vi "Calculate_fit_offset.vi"(0 "baseline1":dbl[](array[numeric]), 3 "baseline2":dbl[](array[numeric])) -> (6 "Peak_ch1":dbl format="%#_6f", 7 "Std_dev_ch1":dbl format="%#_6f", 8 "Peak_ch2":dbl caption="Peak (V)" format="%#_6f", 9 "Std_dev_ch2":dbl caption="Std_dev" format="%#_6f")   [LabVIEW 2019]
uses:
  SiPM_Tests_Global_Var.vi
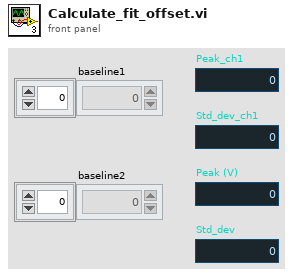
[diagram p1: front panel]
types:
  T1 = cluster{"Numeric Control":dbl, "center":dbl, "standard deviation":dbl, "amplitude":dbl}
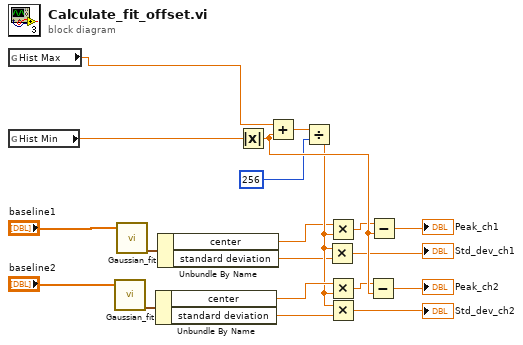
[diagram p0: block diagram]
diagram:
  n1 = global read "SiPM_Tests_Global_Var.vi" "Hist Max"() -> (w2:dbl)
  n2 = global read "SiPM_Tests_Global_Var.vi" "Hist Min"() -> (w1:dbl)
  n3 = call "Gaussian_fit.vi"("Input waveform"="baseline2") -> ("Fit cluster"=w5:T1)  [unwired: 5 in, 1 out]
  n4 = call "Gaussian_fit.vi"("Input waveform"="baseline1") -> ("Fit cluster"=w4:T1)  [unwired: 5 in, 1 out]
  n5 = Unbundle By Name(w5) -> ("center"=w16:dbl, "standard deviation"=w10:dbl)
  n6 = Unbundle By Name(w4) -> ("center"=w12:dbl, "standard deviation"=w9:dbl)
  n7 = Absolute Value(x=w1) -> (abs(x)=w18:dbl)
  n8 = Add(x=w2, y=w18) -> (x+y=w7:dbl)
  n9 = Divide(x=w7, y=256 ("# bins")) -> (x/y=w15:dbl)
  n10 = Multiply(x=w15, y=w9) -> (x*y=→"Std_dev_ch1":dbl)
  n11 = Multiply(x=w12, y=w15) -> (x*y=w13:dbl)
  n12 = Multiply(x=w16, y=w15) -> (x*y=w17:dbl)
  n13 = Multiply(x=w15, y=w10) -> (x*y=→"Std_dev_ch2":dbl)
  n14 = Subtract(x=w17, y=w18) -> (x-y=→"Peak_ch2":dbl)
  n15 = Subtract(x=w13, y=w18) -> (x-y=→"Peak_ch1":dbl)
